vi "CryoStream800.vi"() -> ()   [LabVIEW 2017]
doc: "This example demonstrates how to query an XML document by using an XPath expression and returns all the nodes that match the XPath expression."
panel:
  out "Network":string
  in  "AutoLaunch":bool=TRUE
  out "PhaseStatus":string
  out "iPhaseStatus":i32
  out "Info value":string[](array[string])
  out "Info":string[](array[string])
  in  "Set Temperature (K)":dbl
  out "Gas flow unit":string
  out "Flow":dbl
  out "Back preassure unit":string
  out "Back P":dbl
  out "Suct Temp unit":string
  out "Suct T":dbl format="%_4g"
  out "Evap Temp unit":string
  out "Evap T":dbl format="%_4g"
  out "Suct Heat unit":string
  out "Suct H":dbl format="%#_4g"
  out "Evap Heat unit":string
  out "Evap H":dbl format="%#_4g"
  out "Gas Heat unit":string
  out "Gas H":dbl format="%#_4g"
  out "Valve opening unit":string
  out "Valve":dbl format="%#_4g"
  out "Sample T unit":string
  out "Sample T":dbl format="%_4g"
  out "Alive":bool
  out "DeviceId":string
  out "ConnectionStatus":string
  out "error out 2":errorcluster
  out "iValve":i32
  out "iBackP":i32
  out "iGasFlow":i32
  out "iSuctH":i32
  out "iEvapH":i32
  out "iGasH":i32
  out "iSuctT":i32
  out "iEvapT":i32
  out "iSampleT":i32
  out "Device":string
  out "error out":errorcluster
  in  "stop":bool
  out "value":string[](array[string])
  out "units":string[](array[string])
  out "Properties":string[](array[string])
  # "CRYOSTREAM 800"
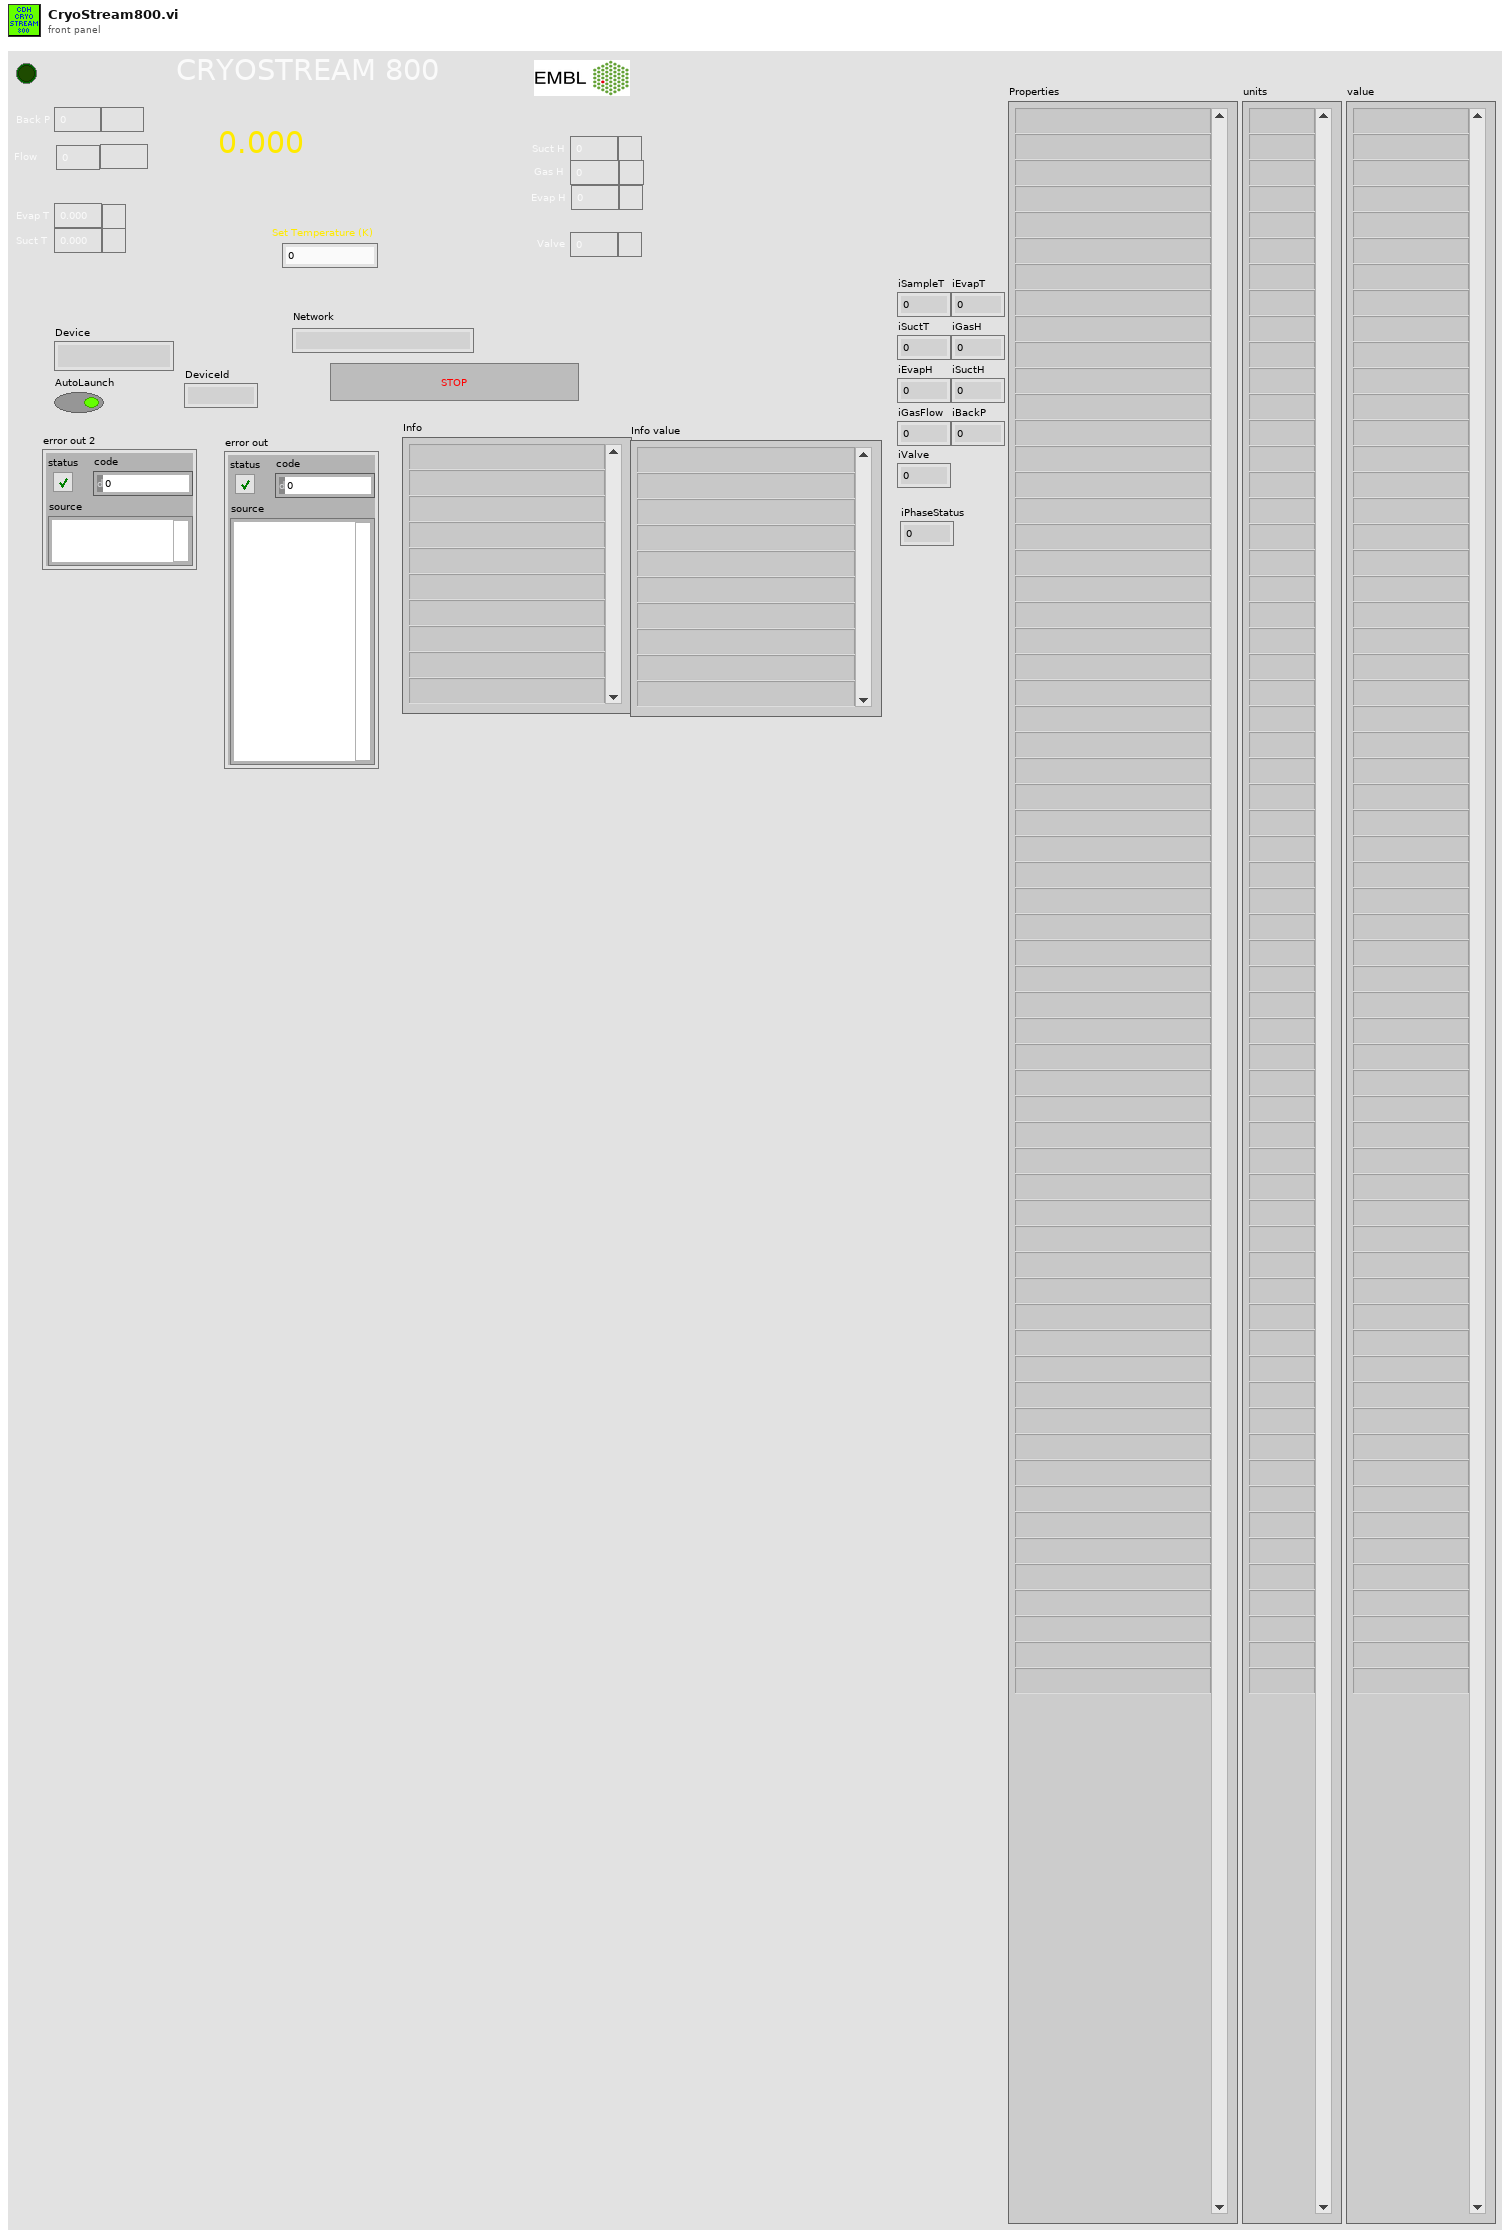
[diagram p1: front panel]
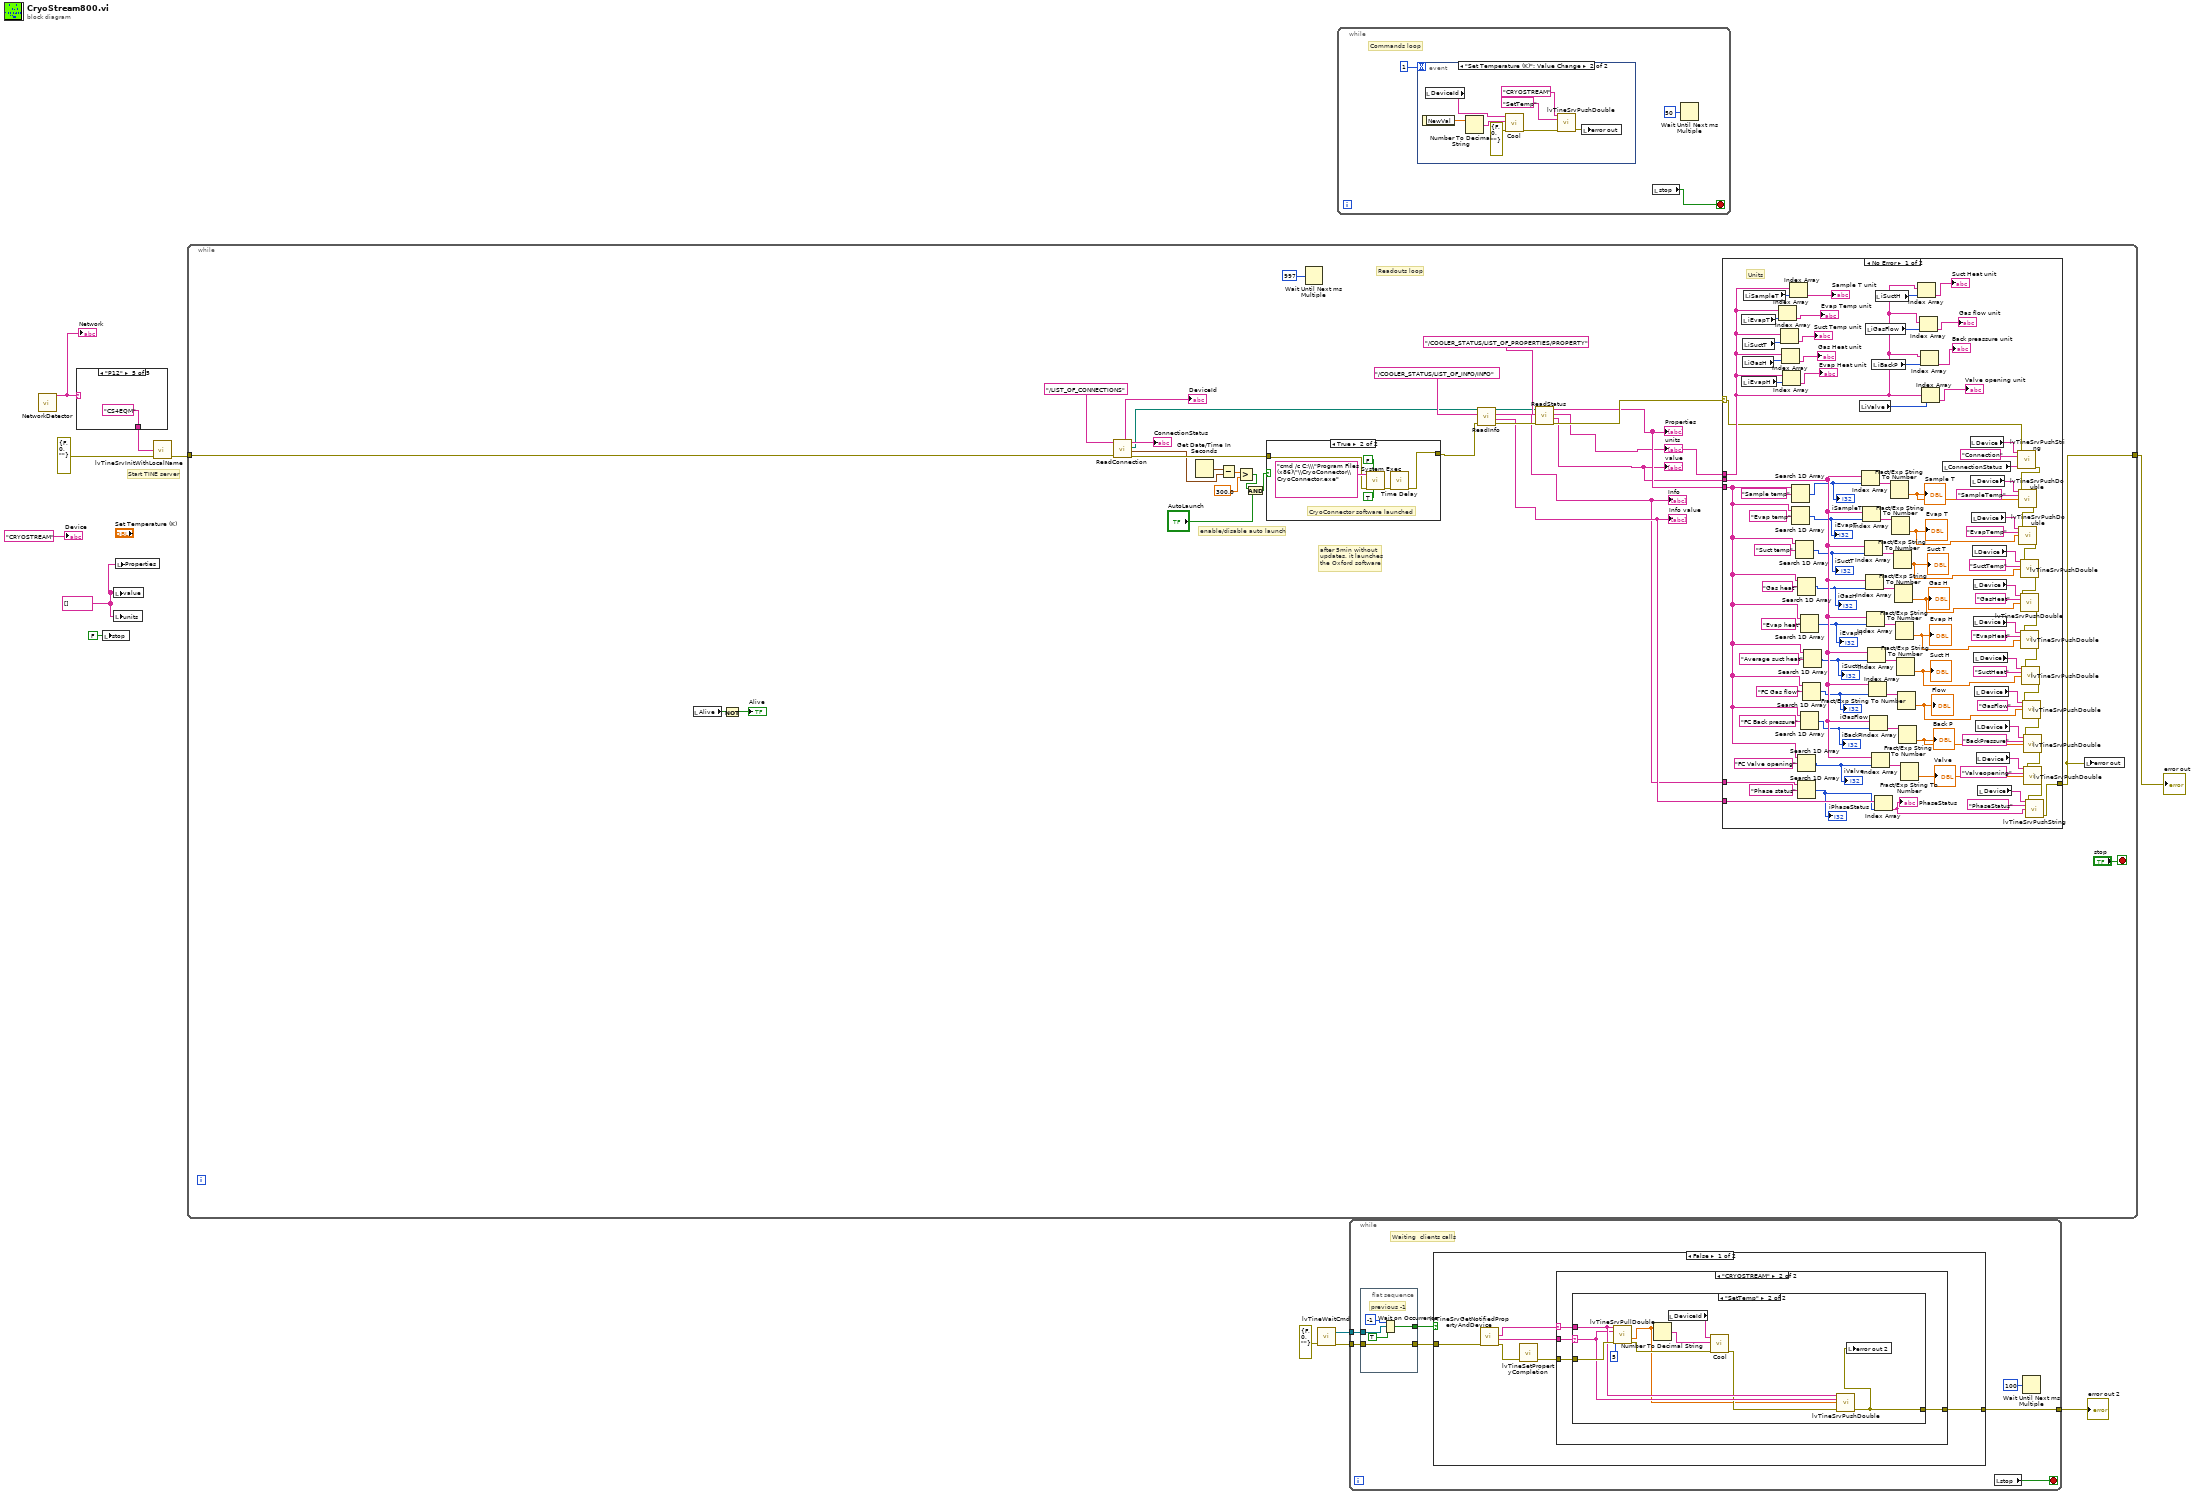
[diagram p0: block diagram]
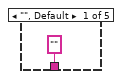
[diagram p2: hidden frame]
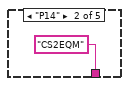
[diagram p3: hidden frame]
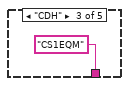
[diagram p4: hidden frame]
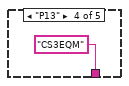
[diagram p5: hidden frame]
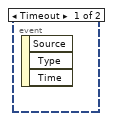
[diagram p6: hidden frame]
diagram:
  w3 = string[] [] ("value")
  # "Start TINE server"
  n1 = call "NetworkDetector.vi"() -> ("Network"=w2:string)  [unwired: 11 in, 4 out]
  "Network" <- w2
  n2 = case shown="\"P12\"" w2 {
    tunnel: ["" ("LocalName") "CS2EQM" ("LocalName") "CS1EQM" ("LocalName") "CS3EQM" ("LocalName") "CS4EQM" ("LocalName")] -> w5
    frame "", Default {
    }
    frame "P14" {
    }
    frame "CDH" {
    }
    frame "P13" {
    }
    frame "P12" {
    }
  }
  n3 = local write "stop"(FALSE ("stop")) -> ()
  n4 = local write "value"(w3) -> ()
  n5 = local write "units"(w3) -> ()
  n6 = local write "Properties"(w3) -> ()
  n7 = call "lvTineSrvInitWithLocalName.vi"("error in (no error)"=errorcluster {"status"=FALSE, "code"=0, "source"=""}, "LocalName"=w5) -> ("error out"=w7:errorcluster)  [unwired: 3 in]
  n8 = while {
    tunnel: w7 -> [w21]
    tunnel: [w36] -> w1
    stop <- "stop" stop-if-true
    # "enable/disable auto launch"
    # "Readouts loop"
    # "after 5min without\nupdates, it launches\nthe Oxford software"
    n9 = local read "Alive"() -> (w41:bool)
    n10 = Not(x=w41) -> (.not. x?=→"Alive":bool)
    n11 = call "ReadConnection.vi"("error in (no error)"=w21, "XPath expression"="/LIST_OF_CONNECTIONS") -> ("error out"=w29:errorcluster, "LastUpdated"=w28:timestamp, "path"=w20:path, "ConnectionStatus"=→"ConnectionStatus":string, "id"=→"DeviceId":string)  [unwired: 5 in]
    n12 = Get Date/Time In Seconds() -> (seconds since 1Jan1904=w44:timestamp)
    n13 = Subtract(x=w44, y=w28) -> (x-y=w43:dbl)
    n14 = Greater?(x=w43, y=300.0) -> (0:w38:bool)
    n15 = And(x=w38, y="AutoLaunch") -> (x .and. y?=w39:bool)
    n16 = case shown="True" w39 {
      tunnel: w29 -> [w145 w147]
      tunnel: [w145 w146] -> w27
      frame False {
      }
      frame True {
        # "CryoConnector software launched"
        n17 = call <vilib>:"System Exec.vi"("run minimized? (F)"=TRUE, "wait until completion? (T)"=FALSE, "error in (no error)"=w147, "command line"="cmd /c C:\\\"Program Files (x86)\"\\CryoConnector\\CryoConnector.exe") -> ("error out"=w148:errorcluster)  [unwired: 4 in, 3 out]
        n18 = call "Time Delay"("error in (no error)"=w148) -> ("error out"=w146:errorcluster)  [unwired: 10 in]
      }
    }
    n19 = Wait Until Next ms Multiple(millisecond multiple=u32 997) -> ()  [unwired: 1 out]
    n20 = call "ReadInfo.vi"("error in (no error)"=w27, "XPath expression"="/COOLER_STATUS/LIST_OF_INFO/INFO", "path to XML document in"=w20) -> ("error out"=w31:errorcluster, "value"=w30:string[], "Info"=w19:string[], "path to XML document out"=w18:path)  [unwired: 4 in]
    "Info" <- w19
    "Info value" <- w30
    n21 = call "ReadStatus.vi"("error in (no error)"=w31, "XPath expression"="/COOLER_STATUS/LIST_OF_PROPERTIES/PROPERTY", "path to XML document"=w18) -> ("error out"=w35:errorcluster, "value"=w32:string[], "units"=w33:string[], "Properties"=w34:string[])  [unwired: 5 in]
    "Properties" <- w34
    "units" <- w33
    "value" <- w32
    n22 = case shown="No Error" w35 {
      selector: w35 -> [w47 w144]
      tunnel: w34 -> [w143 _]
      tunnel: w32 -> [w142 _]
      tunnel: w33 -> [w141 _]
      tunnel: [w140 w144] -> w36
      tunnel: w19 -> [w139 _]
      tunnel: w30 -> [w138 _]
      frame No Error {
        # "Units"
        n23 = local read "iEvapT"() -> (w68:i32)
        n24 = local read "iEvapH"() -> (w71:i32)
        n25 = local read "iSuctT"() -> (w69:i32)
        n26 = local read "iGasH"() -> (w70:i32)
        n27 = local read "iSampleT"() -> (w67:i32)
        n28 = Index Array(array=w141, index=w68) -> (element=→"Evap Temp unit":string)
        n29 = Index Array(array=w141, index=w69) -> (element=→"Suct Temp unit":string)
        n30 = Index Array(array=w141, index=w70) -> (element=→"Gas Heat unit":string)
        n31 = Index Array(array=w141, index=w71) -> (element=→"Evap Heat unit":string)
        n32 = Index Array(array=w141, index=w67) -> (element=→"Sample T unit":string)
        n33 = Search 1D Array(1D array=w143, element="Sample temp") -> (index of element=w84:i32)  [unwired: 1 in]
        "iSampleT" <- w84
        n34 = Search 1D Array(1D array=w143, element="Evap temp") -> (index of element=w83:i32)  [unwired: 1 in]
        "iEvapT" <- w83
        n35 = Search 1D Array(1D array=w143, element="Suct temp") -> (index of element=w82:i32)  [unwired: 1 in]
        "iSuctT" <- w82
        n36 = Search 1D Array(1D array=w143, element="FC Valve opening") -> (index of element=w76:i32)  [unwired: 1 in]
        "iValve" <- w76
        n37 = Search 1D Array(1D array=w139, element="Phase status") -> (index of element=w56:i32)  [unwired: 1 in]
        "iPhaseStatus" <- w56
        n38 = Search 1D Array(1D array=w143, element="Gas heat") -> (index of element=w81:i32)  [unwired: 1 in]
        "iGasH" <- w81
        n39 = Search 1D Array(1D array=w143, element="Evap heat") -> (index of element=w80:i32)  [unwired: 1 in]
        "iEvapH" <- w80
        n40 = Search 1D Array(1D array=w143, element="FC Back pressure") -> (index of element=w77:i32)  [unwired: 1 in]
        "iBackP" <- w77
        n41 = Search 1D Array(1D array=w143, element="FC Gas flow") -> (index of element=w78:i32)  [unwired: 1 in]
        "iGasFlow" <- w78
        n42 = Search 1D Array(1D array=w143, element="Average suct heat") -> (index of element=w79:i32)  [unwired: 1 in]
        "iSuctH" <- w79
        n43 = local read "iValve"() -> (w75:i32)
        n44 = Index Array(array=w142, index=w84) -> (element=w103:string)
        n45 = Index Array(array=w142, index=w83) -> (element=w104:string)
        n46 = Index Array(array=w142, index=w82) -> (element=w105:string)
        n47 = local read "iGasFlow"() -> (w73:i32)
        n48 = Index Array(array=w142, index=w81) -> (element=w106:string)
        n49 = Index Array(array=w142, index=w80) -> (element=w107:string)
        n50 = Index Array(array=w142, index=w79) -> (element=w111:string)
        n51 = Index Array(array=w142, index=w78) -> (element=w110:string)
        n52 = Index Array(array=w142, index=w77) -> (element=w109:string)
        n53 = Index Array(array=w142, index=w76) -> (element=w108:string)
        n54 = local read "iBackP"() -> (w74:i32)
        n55 = Index Array(array=w138, index=w56) -> (element=w53:string)
        "PhaseStatus" <- w53
        n56 = local read "iSuctH"() -> (w72:i32)
        n57 = Fract/Exp String To Number(string=w103) -> (number=w102:dbl)  [unwired: 3 in, 1 out]
        "Sample T" <- w102
        n58 = Fract/Exp String To Number(string=w104) -> (number=w101:dbl)  [unwired: 3 in, 1 out]
        "Evap T" <- w101
        n59 = Fract/Exp String To Number(string=w105) -> (number=w100:dbl)  [unwired: 3 in, 1 out]
        "Suct T" <- w100
        n60 = Fract/Exp String To Number(string=w106) -> (number=w99:dbl)  [unwired: 3 in, 1 out]
        "Gas H" <- w99
        n61 = Fract/Exp String To Number(string=w107) -> (number=w98:dbl)  [unwired: 3 in, 1 out]
        "Evap H" <- w98
        n62 = Fract/Exp String To Number(string=w111) -> (number=w97:dbl)  [unwired: 3 in, 1 out]
        "Suct H" <- w97
        n63 = Fract/Exp String To Number(string=w110) -> (number=w96:dbl)  [unwired: 3 in, 1 out]
        "Flow" <- w96
        n64 = Fract/Exp String To Number(string=w109) -> (number=w95:dbl)  [unwired: 3 in, 1 out]
        "Back P" <- w95
        n65 = Fract/Exp String To Number(string=w108) -> (number=w94:dbl)  [unwired: 3 in, 1 out]
        "Valve" <- w94
        n66 = Index Array(array=w141, index=w72) -> (element=→"Suct Heat unit":string)
        n67 = Index Array(array=w141, index=w73) -> (element=→"Gas flow unit":string)
        n68 = Index Array(array=w141, index=w74) -> (element=→"Back preassure unit":string)
        n69 = Index Array(array=w141, index=w75) -> (element=→"Valve opening unit":string)
        n70 = local read "ConnectionStatus"() -> (w48:string)
        n71 = local read "Device"() -> (w50:string)
        n72 = local read "Device"() -> (w137:string)
        n73 = local read "Device"() -> (w134:string)
        n74 = local read "Device"() -> (w133:string)
        n75 = local read "Device"() -> (w130:string)
        n76 = local read "Device"() -> (w129:string)
        n77 = local read "Device"() -> (w126:string)
        n78 = local read "Device"() -> (w125:string)
        n79 = local read "Device"() -> (w122:string)
        n80 = local read "Device"() -> (w121:string)
        n81 = local read "Device"() -> (w54:string)
        n82 = call "lvTineSrvPushString.vi"("devName"=w50, "prpName"="Connection", "strData"=w48, "error in (no error)"=w47) -> ("error out"=w49:errorcluster)  [unwired: 11 in]
        n83 = call "lvTineSrvPushDouble.vi"("devName"=w137, "prpName"="SampleTemp", "dblData"=w102, "error in (no error)"=w49) -> ("error out"=w119:errorcluster)  [unwired: 11 in]
        n84 = call "lvTineSrvPushDouble.vi"("devName"=w134, "prpName"="EvapTemp", "dblData"=w101, "error in (no error)"=w119) -> ("error out"=w118:errorcluster)  [unwired: 11 in]
        n85 = call "lvTineSrvPushDouble.vi"("devName"=w133, "prpName"="SuctTemp", "dblData"=w100, "error in (no error)"=w118) -> ("error out"=w117:errorcluster)  [unwired: 11 in]
        n86 = call "lvTineSrvPushDouble.vi"("devName"=w130, "prpName"="GasHeat", "dblData"=w99, "error in (no error)"=w117) -> ("error out"=w116:errorcluster)  [unwired: 11 in]
        n87 = call "lvTineSrvPushDouble.vi"("devName"=w129, "prpName"="EvapHeat", "dblData"=w98, "error in (no error)"=w116) -> ("error out"=w115:errorcluster)  [unwired: 11 in]
        n88 = call "lvTineSrvPushDouble.vi"("devName"=w126, "prpName"="SuctHeat", "dblData"=w97, "error in (no error)"=w115) -> ("error out"=w114:errorcluster)  [unwired: 11 in]
        n89 = call "lvTineSrvPushDouble.vi"("devName"=w125, "prpName"="GasFlow", "dblData"=w96, "error in (no error)"=w114) -> ("error out"=w113:errorcluster)  [unwired: 11 in]
        n90 = call "lvTineSrvPushDouble.vi"("devName"=w122, "prpName"="BackPressure", "dblData"=w95, "error in (no error)"=w113) -> ("error out"=w112:errorcluster)  [unwired: 11 in]
        n91 = call "lvTineSrvPushDouble.vi"("devName"=w121, "prpName"="Valveopening", "dblData"=w94, "error in (no error)"=w112) -> ("error out"=w52:errorcluster)  [unwired: 11 in]
        n92 = call "lvTineSrvPushString.vi"("devName"=w54, "prpName"="PhaseStatus", "strData"=w53, "error in (no error)"=w52) -> ("error out"=w140:errorcluster)  [unwired: 11 in]
      }
      frame Error {
      }
    }
    n93 = local write "error out"(w36) -> ()
  }
  "error out" <- w1
  n94 = call "lvTineWaitCmd.vi"("error in (no error)"=errorcluster {"status"=FALSE, "code"=0, "source"=""}) -> ("error out"=w9:errorcluster, "wasCalled"=w8:refnum<k4>)  [unwired: 3 in]
  n95 = while {
    stop <- w153 stop-if-true
    # "Commands loop"
    n96 = event shown="[1] \"Set Temperature (K)\": Value Change" {
      selector: _ -> [_ _]
      dyn-events: _ -> [_ _]
      timeout: 1 -> [_ _]
      event Timeout {
        n97 = event-data() -> ()  [unwired: 1 in, 3 out]
      }
      event "Set Temperature (K)": Value Change {
        n98 = event-data() -> ("NewVal"=w162:dbl)  [unwired: 1 in]
        n99 = local read "DeviceId"() -> (w157:string)
        n100 = Number To Decimal String(number=w162) -> (decimal integer string=w161:string)  [unwired: 1 in]
        n101 = call "Cool.vi"("id"=w157, "Set temp"=w161, "error in (no error)"=errorcluster {"status"=FALSE, "code"=0, "source"=""}) -> ("error out"=w160:errorcluster)  [unwired: 6 in, 1 out]
        n102 = call "lvTineSrvPushDouble.vi"("devName"="CRYOSTREAM", "prpName"="SetTemp", "error in (no error)"=w160) -> ("error out"=w155:errorcluster)  [unwired: 12 in]
        n103 = local write "error out"(w155) -> ()
      }
    }
    n104 = local read "stop"() -> (w153:bool)
    n105 = Wait Until Next ms Multiple(millisecond multiple=u32 50) -> ()  [unwired: 1 out]
  }
  n106 = while {
    tunnel: w8 -> [w169]
    tunnel: w9 -> [w167]
    tunnel: [w164] -> w10
    stop <- w165 stop-if-true
    # "Waiting  clients calls"
    n107 = flat-sequence {
      tunnel: w169 -> [w195]
      tunnel: [w194] -> w168
      tunnel: w167 -> [w193]
      tunnel: [w193] -> w166
      frame #0 {
        # "previous -1"
        n108 = Wait on Occurrence(1:TRUE ("ignore previous (T)"), 2:w195, 3:-1 ("ms timeout (-1)")) -> (0:w194:bool)
      }
    }
    n109 = case shown="False" w168 {
      tunnel: w166 -> [w175 w192]
      tunnel: [w170 w192] -> w164
      frame False {
        n110 = call "lvTineSrvGetNotifiedPropertyAndDevice.vi"("error in (no error)"=w175) -> ("error out"=w174:errorcluster, "CalledPropertyName"=w172:string, "CalledDeviceName"=w173:string)  [unwired: 7 in, 1 out]
        n111 = call "lvTineSetPropertyCompletion.vi"("error in (no error)"=w174) -> ("error out"=w171:errorcluster)  [unwired: 3 in, 1 out]
        n112 = case shown="\"CRYOSTREAM\"" w173 {
          selector: w173 -> [_ w178]
          tunnel: w172 -> [_ w180]
          tunnel: w171 -> [w176 w179]
          tunnel: [w176 w177] -> w170
          frame "False", Default {
          }
          frame "CRYOSTREAM" {
            n113 = case shown="\"SetTemp\"" w180 {
              selector: w180 -> [_ w189]
              tunnel: w179 -> [w181 w191]
              tunnel: w178 -> [_ w190]
              tunnel: [w181 w185] -> w177
              frame "False", Default {
              }
              frame "SetTemp" {
                n114 = call "lvTineSrvPullDouble.vi"("devName"=w190, "prpName"=w189, "Selector for Type"=5 ("stringLength"), "error in (no error)"=w191) -> ("dblData"=w183:dbl, "error out"=w188:errorcluster)  [unwired: 10 in]
                n115 = Number To Decimal String(number=w183) -> (decimal integer string=w184:string)  [unwired: 1 in]
                n116 = local read "DeviceId"() -> (w182:string)
                n117 = call "Cool.vi"("id"=w182, "Set temp"=w184, "error in (no error)"=w188) -> ("error out"=w187:errorcluster)  [unwired: 6 in, 1 out]
                n118 = call "lvTineSrvPushDouble.vi"("devName"=w190, "prpName"=w189, "dblData"=w183, "error in (no error)"=w187) -> ("error out"=w185:errorcluster)  [unwired: 11 in]
                n119 = local write "error out 2"(w185) -> ()
              }
            }
          }
        }
      }
      frame True {
      }
    }
    n120 = local read "stop"() -> (w165:bool)
    n121 = Wait Until Next ms Multiple(millisecond multiple=u32 100) -> ()  [unwired: 1 out]
  }
  "error out 2" <- w10
  "Device" <- "CRYOSTREAM" ("Device")
